vi "Add Result Channels.vi"(8 "error in (no error)":errorcluster, 10 "Selected Waveform Sections items":T1[](array[typedef]) format="%.0x", 11 "RunningAverageCalculation in":refnum<class "RunningAverageCalculation.lvclass">) -> (0 "error out":errorcluster, 3 "RunningAverageCalculation out":refnum<class "RunningAverageCalculation.lvclass">)   [LabVIEW 2015, in "RunningAverageCalculation.lvclass"]
uses:
  RunningAverageCalculation.lvclass
  <vilib>/NI Veristand/Custom Device API/Custom Device Item Ref.ctl
  WaveformCalculation/WaveformCalculation.lvclass/WaveformCalculation.ctl
  <vilib>/NI Veristand/Custom Device API/Custom Device Channel.ctl
  <vilib>/NI Veristand/Custom Device API/Custom Device Channel Type.ctl
  NationalInstruments.VeriStand.SystemStorage
  Shared/Constants.vi
  <vilib>/NI Veristand/Custom Device API/Get Item Property (Dependent Node Pointer).vi
  WaveformCalculation/WaveformCalculation.lvclass
  <vilib>/NI VeriStand/Custom Device API/Custom Device API.lvlib
  Shared/Waveform-Processing-Custom-Device Shared.lvlib
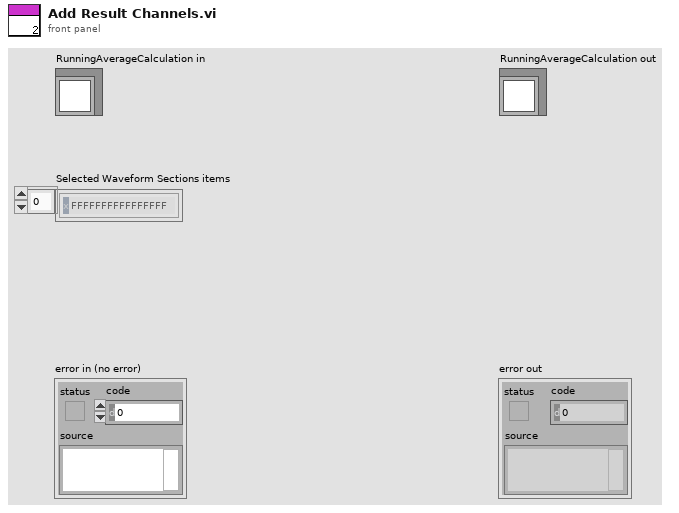
[diagram p1: front panel]
types:
  T1 = typedef "Custom Device API.lvlib/Custom Device Item Ref.ctl" = u64
  T2 = typedef "Custom Device API.lvlib/Custom Device Channel.ctl" = cluster{"Type":T3, "Units":string, "Default Value":dbl, "Faultable":bool, "Scalable":bool}
  T3 = typedef "Custom Device API.lvlib/Custom Device Channel Type.ctl" = enum16{"Input", "Output"}
  T4 = typedef "Custom Device API.lvlib/Custom Device Pointer.ctl" = refnum<k24>
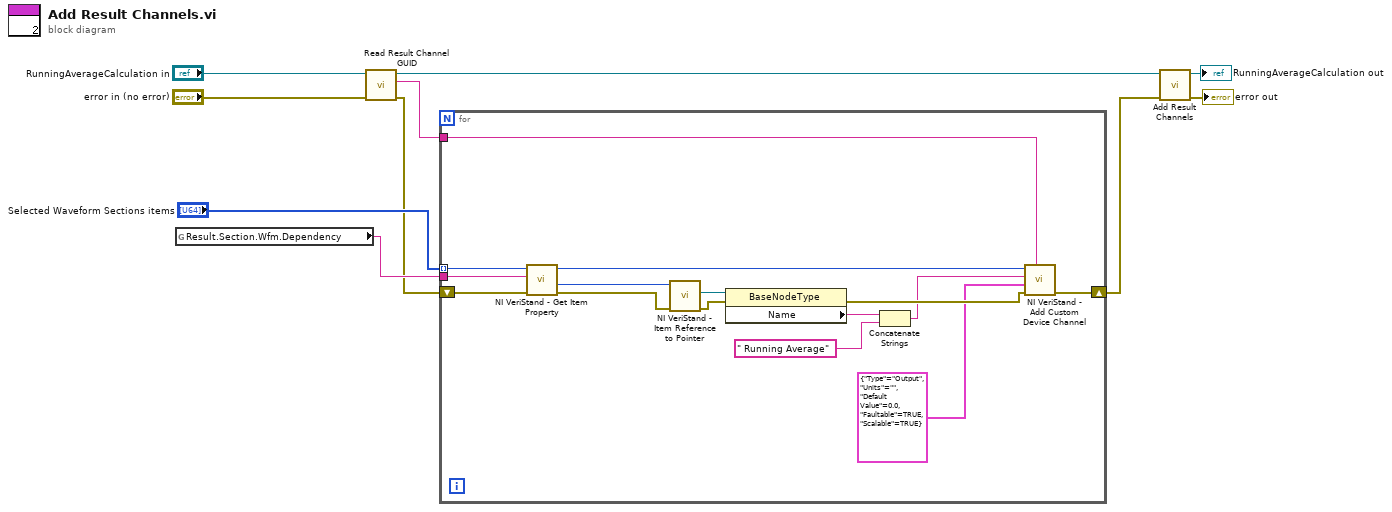
[diagram p0: block diagram]
diagram:
  n1 = global read "Constants.vi" "Result.Section.Wfm.Dependency"() -> (w9:string)
  n2 = call "Read Result Channel GUID.vi"("error in (no error)"="error in (no error)", "WaveformCalculation in"="RunningAverageCalculation in") -> ("error out"=w5:errorcluster, "Result Channel GUID"=w4:string, "WaveformCalculation out"=w2:refnum<class "RunningAverageCalculation.lvclass">)  [unwired: 7 in]
  n3 = for {
    tunnel: w9 -> [w24]
    tunnel: "Selected Waveform Sections items" -> [w23] mode=indexing
    shift-right: [w11] -> w3
    shift-left: w5 -> [w25]
    tunnel: w4 -> [w12]
    n4 = call-poly <vilib>:"NI VeriStand - Get Item Property.vi"("error in (no error)"=w25, "Property Name"=w24, "Item Ref in"=w23) -> ("error out"=w22:errorcluster, "Dependent Node Ref"=w21:T1, "Item Ref out"=w16:T1)  [unwired: 5 in, 1 out]
    n5 = call <vilib>:"NI VeriStand - Item Reference to Pointer.vi"("error in (no error)"=w22, "Item Ref in"=w21) -> ("error out"=w19:errorcluster, "Node Pointer"=w20:T4)  [unwired: 6 in, 2 out]
    n6 = property class="BaseNodeType"(reference=w20, error in=w19) -> (error out=w15:errorcluster, "Name"=w18:string)  [unwired: 1 out]
    n7 = Concatenate Strings(w18, " Running Average" ("string")) -> (w14:string)
    n8 = call <vilib>:"NI VeriStand - Add Custom Device Channel.vi"("GUID (Default Channel)"=w12, "error in (no error)"=w15, "Channel"=T2 {"Type"=enum."Output", "Units"="", "Default Value"=0.0, "Faultable"=TRUE, "Scalable"=TRUE}, "Channel Name"=w14, "Parent Ref in"=w16) -> ("error out"=w11:errorcluster)  [unwired: 3 in, 3 out]
  }
  n9 = call-parent "Add Result Channels.vi"("error in (no error)"=w3, "WaveformCalculation in"=w2) -> ("error out"=→"error out":errorcluster, "WaveformCalculation out"=→"RunningAverageCalculation out":refnum<class "RunningAverageCalculation.lvclass">)  [unwired: 8 in]
